vi "Configure.vi"(8 "error in (no error)":errorcluster) -> (0 "error out":errorcluster, 1 "valid config":bool, 2 "register trends":T1[](array[typedef]), 3 "config":T3[](array[typedef]))   [LabVIEW 2017, in "EmsaAnalysis.lvlib"]
uses:
  <vilib>/addons/InsightCM/Devices/Shared/Emsa/EmsaAnalysis/EmsaAnalysis.lvlib
  <vilib>/addons/InsightCM/Devices/Shared/Emsa/EmsaAnalysis/controls/datagroupMetrics.ctl
  <vilib>/addons/InsightCM/Devices/Shared/Emsa/EmsaAnalysis/controls/channelMetrics.ctl
  <vilib>/addons/InsightCM/Devices/Shared/Emsa/EmsaAnalysis/controls/metric.ctl
  <vilib>/addons/InsightCM/MessageBus/Base/controls/MetricDefinitionInstance.ctl
  <vilib>/addons/InsightCM/MessageBus/Base/controls/KeyValuePair.ctl
  <vilib>/addons/InsightCM/Devices/Shared/Emsa/EmsaAnalysis/controls/sweepInfo.ctl
  <vilib>/addons/InsightCM/Devices/Shared/Common/DataEventCreator/controls/RegisterTrendPoints.ctl
  <vilib>/addons/InsightCM/Devices/Shared/Common/DataEventCreator/controls/Registry_Trend.ctl
  <vilib>/addons/InsightCM/Utilities/GlobalConfiguration/GlobalConfiguration.lvlib
  <vilib>/addons/InsightCM/Utilities/DeviceModelHelpers/DeviceModelHelpers.lvlib
  <vilib>/addons/InsightCM/Devices/Shared/Common/DataEventCreator/DataEventCreator.lvlib
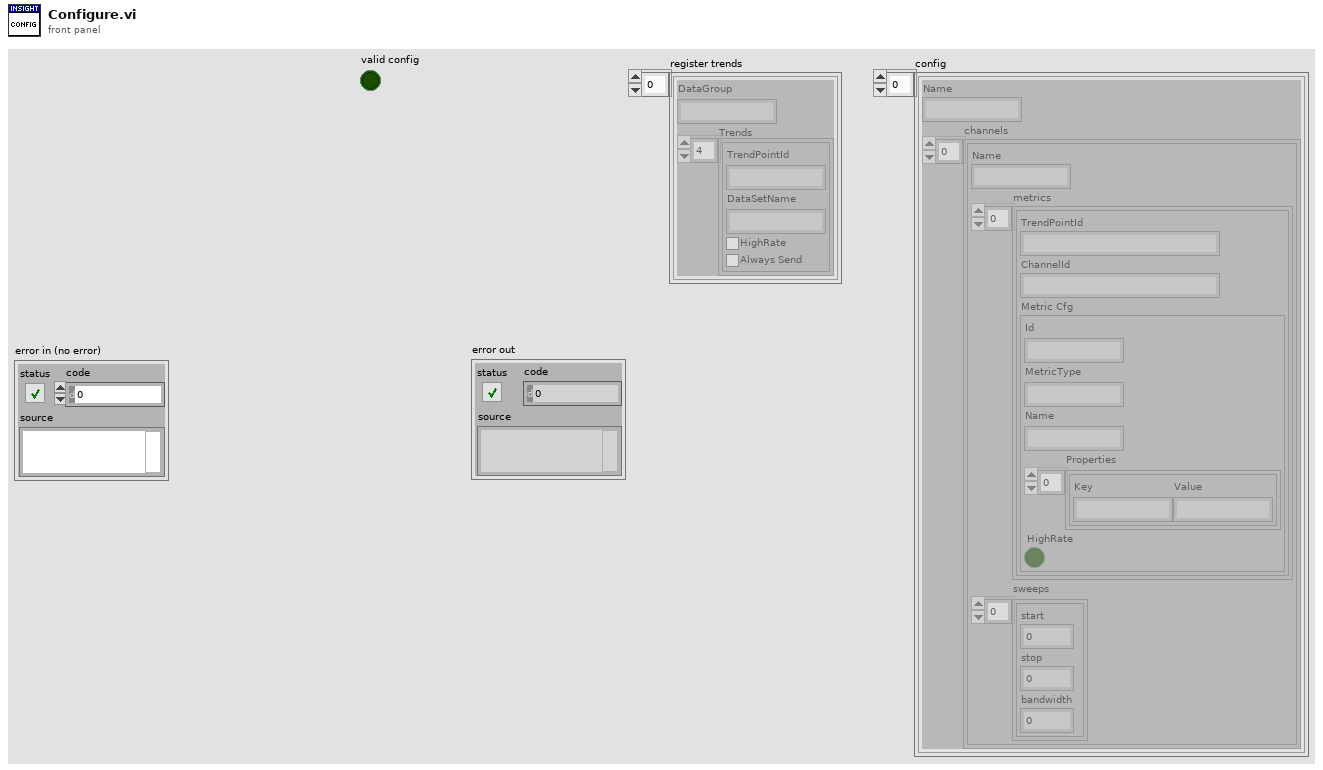
[diagram p1: front panel]
types:
  T1 = typedef "DataEventCreator.lvlib/RegisterTrendPoints.ctl" = cluster{"DataGroup":string, "Trends":T2[]}
  T2 = typedef "DataEventCreator.lvlib/Registry_Trend.ctl" = cluster{"TrendPointId":string, "DataSetName":string, "HighRate":bool, "Always Send":bool}
  T3 = typedef "EmsaAnalysis.lvlib/datagroupMetrics.ctl" = cluster{"Name":string, "channels":T4[]}
  T4 = typedef "EmsaAnalysis.lvlib/channelMetrics.ctl" = cluster{"Name":string, "metrics":T5[], "sweeps":T8[]}
  T5 = typedef "EmsaAnalysis.lvlib/metric.ctl" = cluster{"TrendPointId":string, "ChannelId":string, "Metric Cfg":T6}
  T6 = typedef "MetricDefinitionInstance.ctl" = cluster{"Id":string, "MetricType":string, "Name":string, "Properties":T7[], "HighRate":bool}
  T7 = typedef "KeyValuePair.ctl" = cluster{"Key":string, "Value":string}
  T8 = typedef "EmsaAnalysis.lvlib/sweepInfo.ctl" = cluster{"start":dbl, "stop":dbl, "bandwidth":dbl}
  T9 = typedef "R2_DeviceModel.ctl" = cluster{"Device":T10, "Channels":T17[], "Tags":T19[]}
  T10 = typedef "R2_Device.ctl" = cluster{"Id":string, "Name":string, "DeviceType":string, "HardwareName":string, "IpAddress":string, "HardwareInfo":T7[], "ApplicationType":string, "ApplicationVersion":string, "EquipmentIds":string[], "ConfigurationVersion":string, "State":T11, "Properties":T7[], "DataGroups":T12[], "BurstModeTrigger":T16}
  T11 = typedef "DeviceState.ctl" = cluster{"Disabled":bool}
  T12 = typedef "R2_DataGroup.ctl" = cluster{"Name":string, "OperatingStates":T13[], "Properties":T7[], "EquipmentIds":string[], "AssetNodeId":string}
  T13 = typedef "OperatingState.ctl" = cluster{"Name":string, "Properties":T7[], "Triggers":T14[]}
  T14 = typedef "Trigger.ctl" = cluster{"Type":string, "Expression":string, "Conditions":T15[]}
  T15 = typedef "Condition.ctl" = cluster{"Source":string, "Type":string, "Operator":string, "CompareTo":string, "DwellSeconds":dbl}
  T16 = typedef "BurstModeTrigger.ctl" = cluster{"Trigger":T14, "SampleRate":string, "AcquisitionLength":string}
  T17 = typedef "R2_Channel.ctl" = cluster{"Id":string, "DeviceId":string, "Name":string, "ChannelType":string, "HardwareKey":string, "HardwareChannel":string, "DataGroup":string, "Keywords":string[], "EquipmentIds":string[], "Properties":T7[], "Metrics":T18[], "AssetNodeId":string, "MeasType":string, "AssetName":string}
  T18 = typedef "Metric.ctl" = cluster{"Id":string, "Name":string, "Unit":string, "Properties":T7[], "MetricDefinitionInstanceId":string}
  T19 = typedef "Tag.ctl" = cluster{"Id":string, "Path":string, "Name":string, "Datatype":string, "Props":T7[], "Keywords":string[]}
  T20 = typedef "AssetNode.ctl" = cluster{"Id":string, "Type":string, "Name":string, "ParentIds":string[], "State":T21, "MeasType":string, "Properties":T7[], "OperatingStates":T13[], "Metrics":T18[], "TrendAlarmRules":T22[], "References":T25[]}
  T21 = typedef "AssetState.ctl" = cluster{"Disabled":bool}
  T22 = typedef "TrendAlarmRule.ctl" = cluster{"Id":string, "AssetNodeId":string, "TrendId":string, "Disabled":bool, "OperatingState":string, "Operator":string, "Hysteresis":dbl, "OnDelaySeconds":dbl, "OffDelaySeconds":dbl, "Levels":T23[], "Properties":T7[]}
  T23 = typedef "TrendAlarmLevel.ctl" = cluster{"Severity":i32, "CompareTo":dbl, "Actions":T24[]}
  T24 = typedef "AlarmAction.ctl" = cluster{"Type":string, "Props":T7[]}
  T25 = typedef "AssetNodeReference.ctl" = cluster{"NodeId":string, "Name":string}
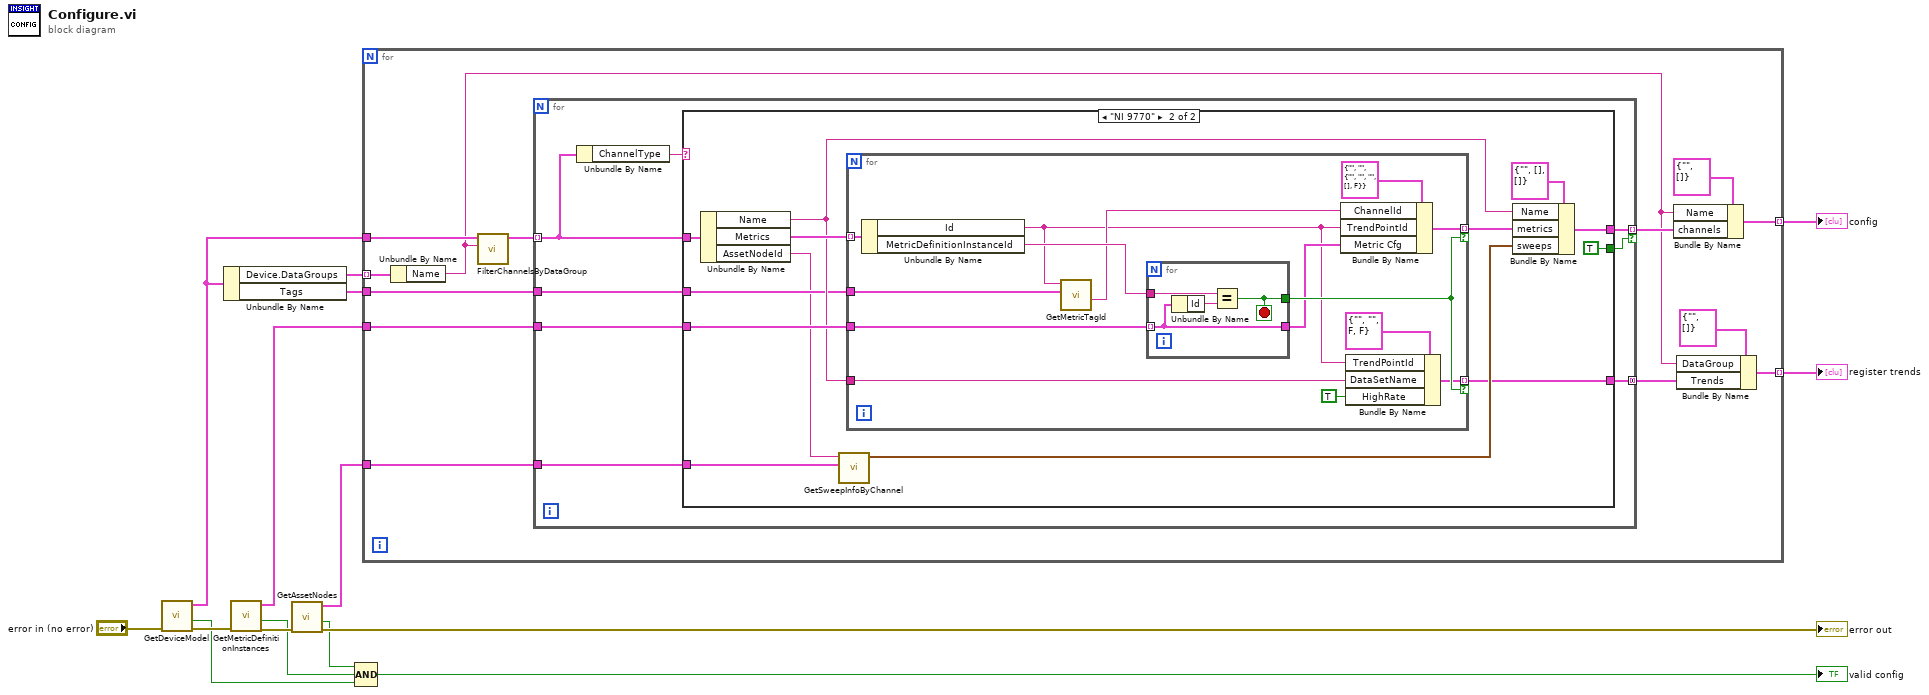
[diagram p0: block diagram]
diagram:
  n1 = call <vilib>:"GetDeviceModel.vi"("error in (no error)"="error in (no error)") -> ("error out"=w6:errorcluster, "found"=w2:bool, "device model"=w9:T9)  [unwired: 8 in]
  n2 = Unbundle By Name(w9) -> ("Device.DataGroups"=w14:T12[], "Tags"=w11:T19[])
  n3 = call <vilib>:"GetMetricDefinitionInstances.vi"("error in (no error)"=w6) -> ("error out"=w7:errorcluster, "found"=w3:bool, "metrics"=w13:T6[])  [unwired: 8 in]
  n4 = call <vilib>:"GetAssetNodes.vi"("error in (no error)"=w7) -> ("error out"=→"error out":errorcluster, "found"=w4:bool, "AssetNodes"=w10:T20[])  [unwired: 8 in]
  n5 = Compound Arithmetic op=AND(w4, w3, w2) -> (→"valid config":bool)
  n6 = for {
    tunnel: w14 -> [w28] mode=indexing
    tunnel: w9 -> [w27]
    tunnel: w13 -> [w26]
    tunnel: [w25] -> w8 mode=indexing
    tunnel: [w21] -> w12 mode=indexing
    tunnel: w11 -> [w20]
    tunnel: w10 -> [w18]
    n7 = Unbundle By Name(w28) -> ("Name"=w23:string)
    n8 = call <vilib>:"FilterChannelsByDataGroup.vi"("group"=w23, "device model"=w27) -> ("channels in data group"=w19:T17[])  [unwired: 8 in, 1 out]
    n9 = for {
      tunnel: w19 -> [w36] mode=indexing
      tunnel: w26 -> [w35]
      tunnel: [w34] -> w24 mode=indexing if=w33
      tunnel: w20 -> [w32]
      tunnel: w18 -> [w31]
      tunnel: [w29] -> w16 mode=concatenating
      n10 = Unbundle By Name(w36) -> ("ChannelType"=w30:string)
      n11 = case shown="\"NI 9770\"" w30 {
        tunnel: w36 -> [_ w49]
        tunnel: w35 -> [_ w47]
        tunnel: [_ w43] -> w34
        tunnel: [_ TRUE] -> w33
        tunnel: w32 -> [_ w41]
        tunnel: w31 -> [_ w39]
        tunnel: [_ w37] -> w29
        frame "", Default {
        }
        frame "NI 9770" {
          n12 = Unbundle By Name(w49) -> ("Name"=w45:string, "Metrics"=w48:T18[], "AssetNodeId"=w38:string)
          n13 = call <vilib>:"GetSweepInfoByChannel.vi"("AssetNodes"=w39, "AssetNodeId"=w38) -> ("sweeps"=w40:T8[])  [unwired: 9 in]
          n14 = for {
            tunnel: w48 -> [w63] mode=indexing
            tunnel: w47 -> [w61]
            tunnel: [w54] -> w37 mode=indexing if=w58
            tunnel: w45 -> [w51]
            tunnel: [w59] -> w46 mode=indexing if=w58
            tunnel: w41 -> [w57]
            n15 = Unbundle By Name(w63) -> ("Id"=w50:string, "MetricDefinitionInstanceId"=w62:string)
            n16 = call <vilib>:"GetMetricTagId.vi"("tags"=w57, "metric id"=w50) -> ("tag id"=w53:string)  [unwired: 7 in, 2 out]
            n17 = for {
              tunnel: w62 -> [w67]
              tunnel: w61 -> [w65] mode=indexing
              tunnel: [w65] -> w56
              tunnel: [w64] -> w58
              stop <- w64 stop-if-true
              n18 = Unbundle By Name(w65) -> ("Id"=w66:string)
              n19 = Equal?(x=w67, y=w66) -> (x = y?=w64:bool)
            }
            n20 = Bundle By Name(cluster=T5 {"TrendPointId"="", "ChannelId"="", "Metric Cfg"={"Id"="", "MetricType"="", "Name"="", "Properties"=[], "HighRate"=FALSE}}, "ChannelId"=w53, "TrendPointId"=w50, "Metric Cfg"=w56) -> (w59:T5)
            n21 = Bundle By Name(cluster=T2 {"TrendPointId"="", "DataSetName"="", "HighRate"=FALSE, "Always Send"=FALSE} ("Trend"), "TrendPointId"=w50, "DataSetName"=w51, "HighRate"=TRUE) -> (w54:T2)
          }
          n22 = Bundle By Name(cluster=T4 {"Name"="", "metrics"=[], "sweeps"=[]} ("channel metrics"), "Name"=w45, "metrics"=w46, "sweeps"=w40) -> (w43:T4)
        }
      }
    }
    n23 = Bundle By Name(cluster=T3 {"Name"="", "channels"=[]} ("datagroup metrics"), "Name"=w23, "channels"=w24) -> (w21:T3)
    n24 = Bundle By Name(cluster=T1 {"DataGroup"="", "Trends"=[]} ("register trend"), "DataGroup"=w23, "Trends"=w16) -> (w25:T1)
  }
  "config" <- w12
  "register trends" <- w8
